vi "Transcriptor LabVIEW to C code Composer.vi"(8 "error in (no error)":errorcluster, 11 "C code Composer Cluster in":T1) -> (0 "error out":errorcluster, 2 "transcripted code":string, 3 "output cluster":T3)   [LabVIEW 2014]
uses:
  types/LabVIEW Universal Transcriptor Cluster.ctl
  types/LabVIEW Universal Transcriptor C code Composer Input Cluster.ctl
  types/LabVIEW Universal Transcriptor Structure Definitions.ctl
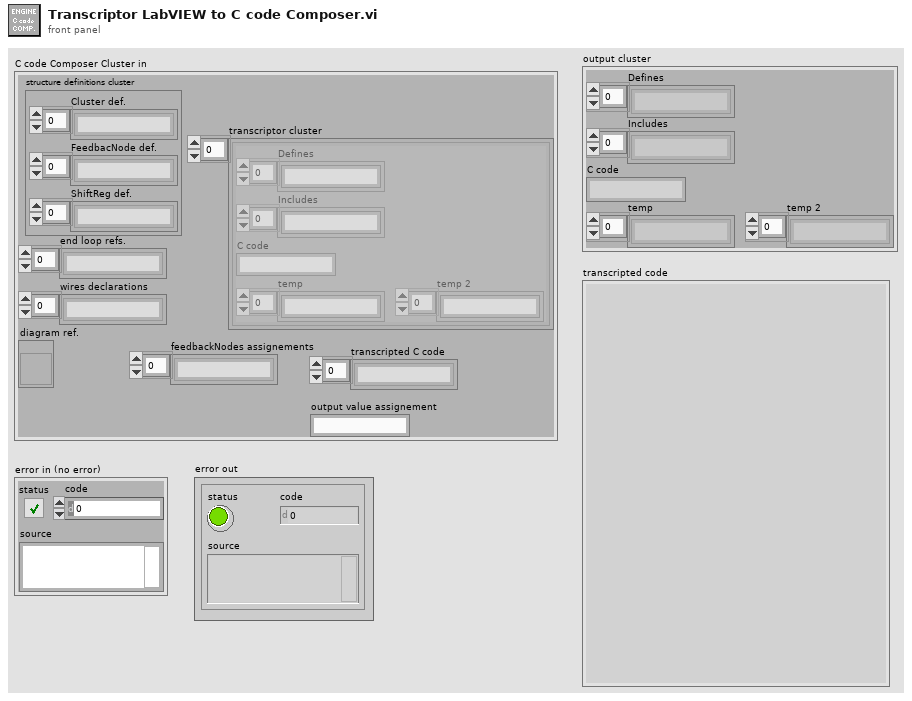
[diagram p1: front panel]
types:
  T1 = typedef "LabVIEW Universal Transcriptor C code Composer Input Cluster.ctl" = cluster{"structure definitions cluster":T2, "end loop refs.":string[], "wires declarations":string[], "diagram ref.":refnum<vi>, "transcriptor cluster":T3[], "transcripted C code":string[], "output value assignement":string, "feedbackNodes assignements":string[]}
  T2 = typedef "LabVIEW Universal Transcriptor Structure Definitions.ctl" = cluster{"Cluster def.":string[], "FeedbacNode def.":string[], "ShiftReg def.":string[]}
  T3 = typedef "LabVIEW Universal Transcriptor Cluster.ctl" = cluster{"Defines":string[], "Includes":string[], "C code":string, "temp":string[], "temp 2":string[]}
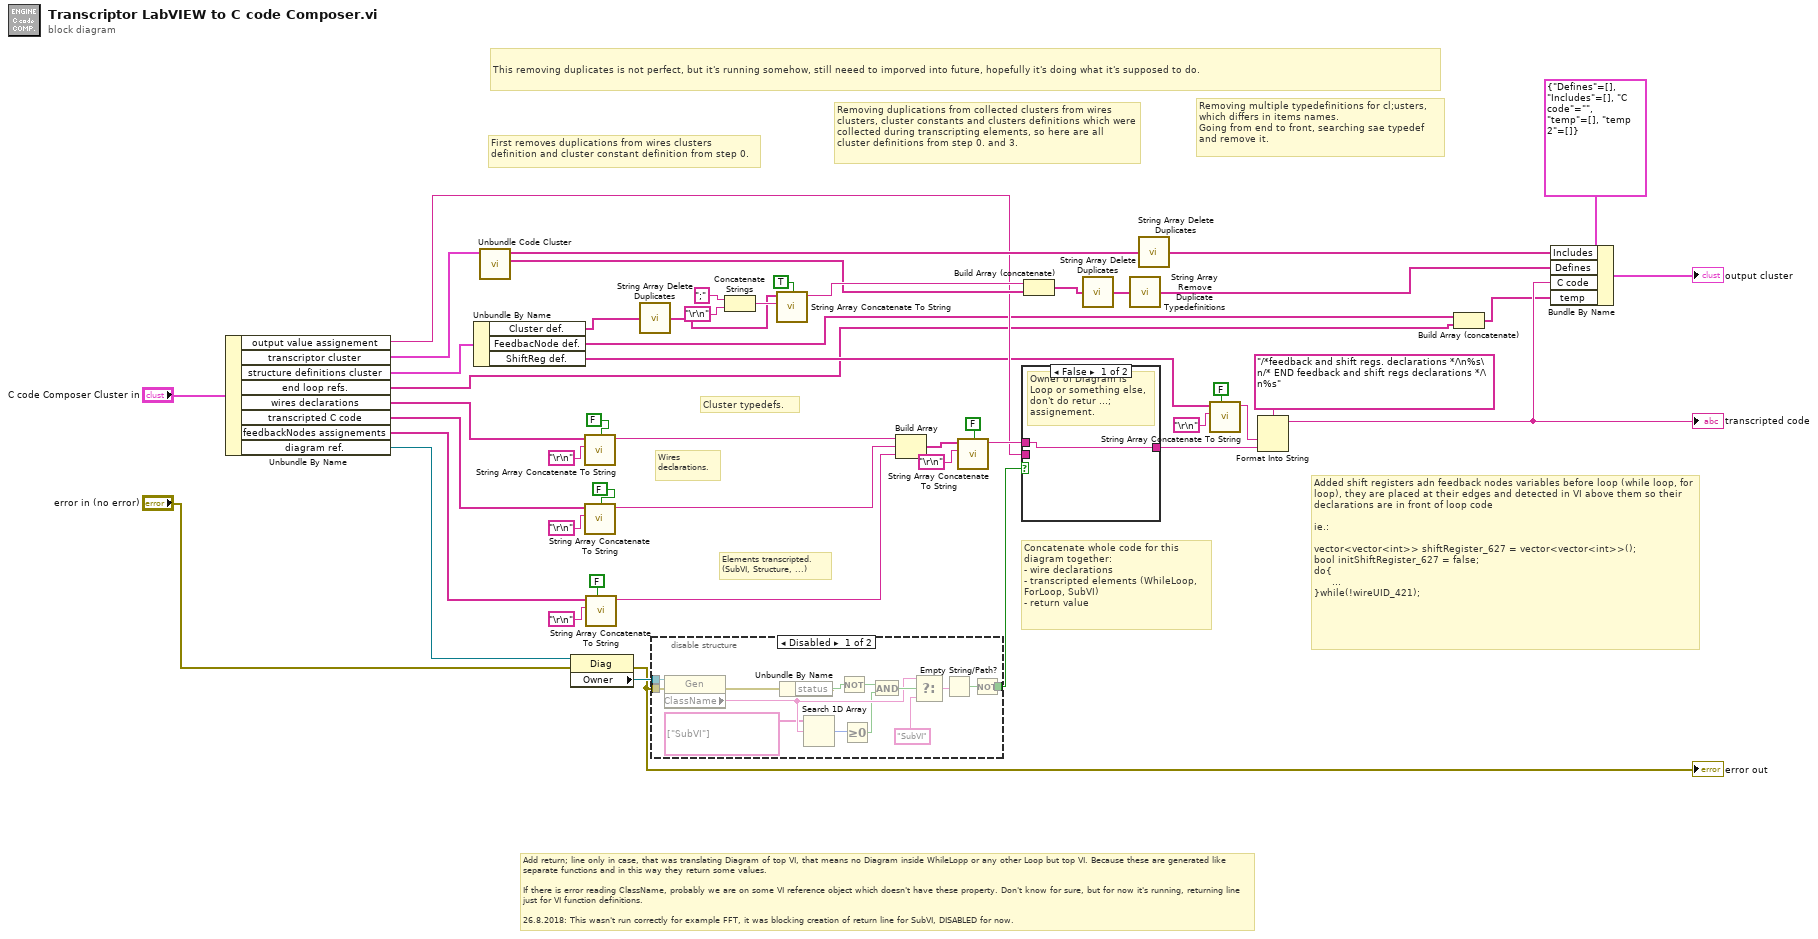
[diagram p0: block diagram]
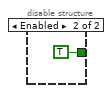
[diagram p2: hidden frame]
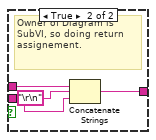
[diagram p3: hidden frame]
diagram:
  # "This removing duplicates is not perfect, but it's running somehow, still neeed to imporved into future, hopefully it's doing what it's supposed to do."
  # "Removing duplications from collected clusters from wires clusters, cluster constants and clusters definitions which were collected during transcripting elements, so here are all cluster definitions from step 0. and 3."
  # "First removes duplications from wires clusters definition and cluster constant definition from step 0."
  # "Added shift registers adn feedback nodes variables before loop (while loop, for loop), they are placed at their edges and detected in VI above them so their declarations are in front of loop code\n\nie.:\n\nvector<vector<int>> shiftRegister_627 = vector<vector<int>>();\nbool initShiftRegister_627 = false;\ndo{\n      ...\n}while(!wireUID_421);"
  # "Removing multiple typedefinitions for cl;usters, which differs in items names.\nGoing from end to front, searching sae typedef and remove it."
  # "Add return; line only in case, that was translating Diagram of top VI, that means no Diagram inside WhileLopp or any other Loop but top VI. Because these are generated like separate functions and in this way they return some values.\n\nIf there is error reading ClassName, probably we are on some VI reference object which doesn't have these property. Don't know for sure, but for now it's running, returning line just for VI function definitions.\n\n26.8.2018: This wasn't run correctly for example FFT, it was blocking creation of return line for SubVI, DISABLED for now."
  # "Concatenate whole code for this diagram together:\n- wire declarations\n- transcripted elements (WhileLoop, ForLoop, SubVI)\n- return value"
  # "Elements transcripted.\n(SubVI, Structure, ...)"
  # "Wires declarations."
  # "Cluster typedefs."
  n1 = Unbundle By Name("C code Composer Cluster in") -> ("output value assignement"=w26:string, "transcriptor cluster"=w25:T3[], "structure definitions cluster"=w24:T2, "end loop refs."=w6:string[], "wires declarations"=w23:string[], "transcripted C code"=w22:string[], "feedbackNodes assignements"=w21:string[], "diagram ref."=w20:refnum<vi>)
  n2 = Unbundle By Name(w24) -> ("Cluster def."=w2:string[], "FeedbacNode def."=w5:string[], "ShiftReg def."=w7:string[])
  n3 = call "Unbundle Code Cluster.vi"("code chunks cluster"=w25) -> ("Defines"=w37:string[], "Includes"=w44:string[])  [unwired: 7 in, 2 out]
  n4 = property class="Diag"(reference=w20, error in="error in (no error)") -> (error out=w18:errorcluster, "Owner"=w39:refnum<vi>)  [unwired: 1 out]
  "error out" <- w18
  n5 = call "String Array Concatenate To String.vi"("insert last delimiter?"=FALSE, "Delimiter char"="\r\n", "Array String In"=w23) -> ("String"=w46:string)  [unwired: 8 in]
  n6 = call "String Array Concatenate To String.vi"("insert last delimiter?"=FALSE, "Delimiter char"="\r\n", "Array String In"=w22) -> ("String"=w47:string)  [unwired: 8 in]
  n7 = call "String Array Concatenate To String.vi"("insert last delimiter?"=FALSE, "Delimiter char"="\r\n", "Array String In"=w21) -> ("String"=w50:string)  [unwired: 8 in]
  n8 = call "String Array Delete Duplicates.vi"("Array"=w2) -> ("Output array"=w1:string[])
  n9 = disable-structure shown="Disabled" {
    disable-tunnel: w39 -> [w56 _]
    disable-tunnel: w18 -> [w54 _]
    disable-tunnel: [w51 TRUE] -> w3
    frame Disabled {
      n10 = property class="Gen"(reference=w56, error in=w54) -> (error out=w55:errorcluster, "ClassName"=w62:string)  [unwired: 1 out]
      n11 = Unbundle By Name(w55) -> ("status"=w61:bool)
      n12 = Search 1D Array(1D array=string[] ["SubVI"], element=w62) -> (index of element=w59:i32)  [unwired: 1 in]
      n13 = Not(x=w61) -> (.not. x?=w57:bool)
      n14 = Greater Or Equal To 0?(x=w59) -> (x >= 0?=w60:bool)
      n15 = And(x=w57, y=w60) -> (x .and. y?=w64:bool)
      n16 = Select(t=w62, s=w64, f="SubVI") -> (s? t:f=w52:string)
      n17 = Empty String/Path?(string/path=w52) -> (empty?=w53:bool)
      n18 = Not(x=w53) -> (.not. x?=w51:bool)
    }
    frame Enabled {
    }
  }
  n19 = Concatenate Strings(";" ("string"), "\r\n") -> (w42:string)
  n20 = call "String Array Concatenate To String.vi"("insert last delimiter?"=TRUE, "Delimiter char"=w42, "Array String In"=w1) -> ("String"=w43:string)  [unwired: 8 in]
  n21 = Build Array(w46, w47, w50) -> (w33:string[])
  n22 = call "String Array Concatenate To String.vi"("insert last delimiter?"=FALSE, "Delimiter char"="\r\n", "Array String In"=w33) -> ("String"=w38:string)  [unwired: 8 in]
  n23 = case shown="False" w3 {
    tunnel: w38 -> [w66 w70]
    tunnel: [w66 w69] -> w13
    tunnel: w26 -> [_ w68]
    frame False {
      # "Owner of Diagram is Loop or something else, don't do retur ...; assignement."
    }
    frame True {
      # "Owner of Diagram is SubVI, so doing return assignement."
      n24 = Concatenate Strings(w70, "\r\n", w68) -> (w69:string)
    }
  }
  n25 = Build Array (concatenate)(w43, w37) -> (w16:string[])
  n26 = call "String Array Delete Duplicates.vi"("Array"=w16) -> ("Output array"=w15:string[])
  n27 = call "String Array Remove Duplicate Typedefinitions.vi"("Array"=w15) -> ("Output array"=w14:string[])
  n28 = call "String Array Delete Duplicates.vi"("Array"=w44) -> ("Output array"=w17:string[])
  n29 = call "String Array Concatenate To String.vi"("insert last delimiter?"=FALSE, "Delimiter char"="\r\n", "Array String In"=w7) -> ("String"=w8:string)  [unwired: 8 in]
  n30 = Format Into String(format string="/*feedback and shift regs. declarations */\n%s\n/* END feedback and shift regs declarations */\n%s", w8, w13) -> (resulting string=w12:string)  [unwired: 2 in, 1 out]
  "transcripted code" <- w12
  n31 = Build Array (concatenate)(w5, w6) -> (w4:string[])
  n32 = Bundle By Name(cluster=T3 {"Defines"=[], "Includes"=[], "C code"="", "temp"=[], "temp 2"=[]} ("input cluster"), "Includes"=w17, "Defines"=w14, "C code"=w12, "temp"=w4) -> (→"output cluster":T3)
